vi "LIA Debugging Slow Host.vi"() -> ()   [LabVIEW 2017]
uses:
  Program Files (x86)/National Instruments/LabVIEW 2017/examples/Lock-In Amplifier/lib/host/Public/pll settings.ctl
  Program Files (x86)/National Instruments/LabVIEW 2017/examples/Lock-In Amplifier/lib/host/Public/lock-in settings.ctl
  Slow Class/LIA Debugging Slow.lvclass
  C:/Repositories/Lock-In-Amplifier/Debugging/Class/LIA Debugging.lvclass
  C:/Program Files (x86)/National Instruments/LabVIEW 2017/examples/Lock-In Amplifier/lib/interface/Interface/LIA Host Interface.lvclass
  <vilib>/measure/maspectr.llb/Power Spectrum and PSD Export Mode.ctl
  <vilib>/addons/Digital Filter Design/Analysis.llb/DFD Plot Freq Response (Linear-Spaced).vi
  <vilib>/measure/maspectr.llb/FFT Power Spectrum and PSD for N Chan.vi
  <vilib>/Utility/error.llb/Error Cluster From Error Code.vi
  <vilib>/rvi/errors/niLvFpgaAdjustHostInterfaceError.vi
  <vilib>/rvi/interface/nirviReadWriteControl/nirviReadWriteControl.xnode
  Program Files (x86)/National Instruments/LabVIEW 2017/examples/Lock-In Amplifier/lib/host/Lock-In Amplifier Example Host.lvlib
  Class/LIA Debugging.lvclass
  <vilib>/measure/NI_MAPro.lvlib
  <vilib>/addons/Digital Filter Design/NI_DigFilterLicensed.lvlib
  NiFpgaLv.dll
  <vilib>/rvi/interface/Simulation/niFpgaSimulationCallBeginRW.vi
  <vilib>/Analysis/4window.llb/windowTd.ctl
  <vilib>/Analysis/NI_AALPro.lvlib
  <vilib>/Analysis/NI_AALBase.lvlib
  <vilib>/measure/maspectr.llb/FFT Power Spectrum and PSD for 1 Chan (CDB).vi
panel:
  in  "Tab Control 2":enum32{"Page 1", "Page 2"}(tab)
  in  "restart averaging (F)":bool
  in  "dpll.m 0":i8=-20
  in  "lock-in.decimator0 0":enum16{"None", "CIC", "FIR", "2x4HB", "2x4SOS"}(ring)=enum."FIR"
  in  "averaging parameters":T1={"averaging mode"=enum."RMS averaging", "weighting mode"=enum."Exponential", "number of averages"=10} {"number of averages" min=1}
  in  "Host decimation?":bool
  in  "lock-in.iir config 0":T2={"b0"=0.001556396484375, "b1"=-0.000762939453125, "-a1"=1.9305267333984375, "-a2"=-0.9328765869140625} {"b0" format="%.17g"; "b1" format="%.17g"; "-a1" format="%.17g"; "-a2" format="%.17g"}
  out "lock-in.max-min":dbl=1.9775797561733533e-07 caption="Deviation" format="%#_6p"
  out "lock-in.min":dbl=1.9775797561733533e-07 caption="Deviation" format="%#_6p"
  out "lock-in.max":dbl=1.9775797561733533e-07 caption="Deviation" format="%#_6p"
  in  "Tab Control 1":T3(tab)
  out "pll.vco output 0":fxp<+/-,48,0> format="%#.18g"
  out "lock-in.cic config 0":cluster{"factor":fxp<+,16,16>, "shift":i16}
  out "dpll.vco output 0":fxp<+/-,48,0> format="%#.18g"
  out "dpll.config 0":T4
  out "nco.frequency 0":fxp<+/-,48,0>=0.0010000000000012221 format="%#_19g"
  out "stream.state 0":T5(ring)
  out "size(s) 1":i32
  out "lock-in.carrier 0 read":fxp<+/-,48,0> format="%_19g"
  out "stream.overflow? 0":bool
  out "size(s) 2":i32
  out "lock-in.decimator0 0 read":enum16{"None", "CIC", "FIR", "2x4HB", "2x4SOS"}(ring)
  out "size(s) 3":i32
  out "# elements in queue":i32
  out "Power Spectrum (dBm)":cluster{"f0":dbl, "df":dbl, "magnitude":dbl[]}[](graph)
  out "Waveform Graph 3":dbl[][](graph)
  out "Waveform Graph 4":dbl[][](graph)
  out "Waveform Graph 6":waveform(dbl)[](graph)
  out "Waveform Graph 2":cluster{"f0":dbl, "df":dbl, "values":dbl[]}[](graph)
  out "Waveform Graph":cluster{"f0":dbl, "df":dbl, "magnitude":dbl[]}[](graph)
  in  "app.quit":bool
  in  "lock-in.record length 0":u32=2048 caption="Record Length"
  in  "app.tab 0":enum32{"Lock-In", "PLL", "Output"}(tab)
  in  "lock-in.sampling rate":dbl=100000000.0 caption="Sampling Rate" format="%_10p"
  in  "lock-in.decimation0 0":i32=256 caption="Decimation 0"
  in  "lock-in.source 0":enum16{"AI 0", "AI 1", "AI 2", "AI 3", "NCO 0"}(ring)=enum."AI 1" caption="Channel"
  in  "lock-in.carrier 0":T6(ring)=enum."DPLL 0" caption="Carrier Source"
  in  "lock-in.manual carrier 0":dbl=100000.0 caption="Carrier Frequency" format="%_10p"
  in  "pll.source 0":enum16{"AI 0", "AI 1", "AI 2", "AI 3"}(ring) caption="Source"
  in  "pll.q frequency 0":dbl=100000.0 caption="Q Frequency" format="%#_6p"
  in  "pll.reset 0":bool caption="PLL Reset"
  in  "ao.level 0":dbl=0.5 caption="AO 0 Level" format="%#_6pV"
  in  "ao.frequency 0":dbl=10000000.0 caption="AO 0 Frequency" format="%#.9p"
  in  "rio device":tag="PXI2Slot2" caption="Resource"
  out "lock-in.deviation":dbl=1.9775797561733533e-07 caption="Deviation" format="%#_6p"
  out "lock-in.mean":dbl=8.221341747482856e-05 format="%#_12p"
  out "Result":cluster{dbl, "standard deviation":dbl}(graph)
  # "NI Lock-In Amplifier Reference Example"
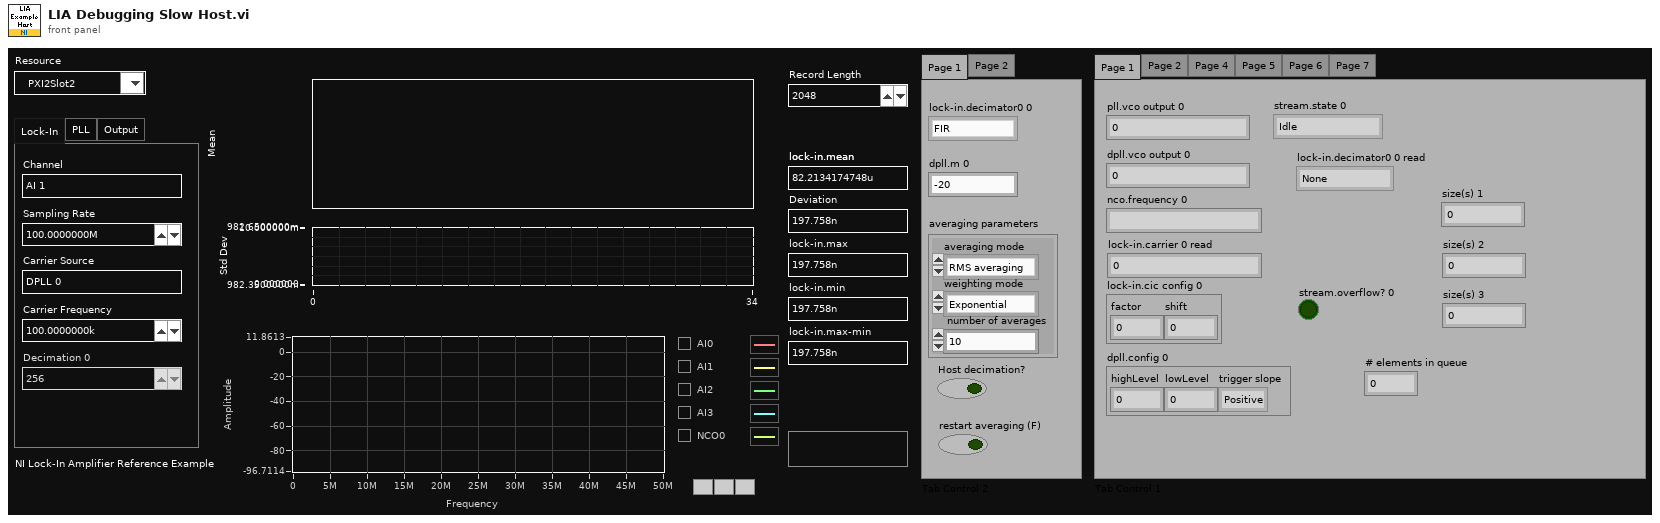
[diagram p1: front panel]
types:
  T1 = cluster{"averaging mode":enum16{"No averaging", "Vector averaging", "RMS averaging", "Peak hold"}, "weighting mode":enum16{"Linear", "Exponential"}, "number of averages":u32}
  T2 = cluster{"b0":fxp<+/-,18,2>, "b1":fxp<+/-,18,2>, "-a1":fxp<+/-,18,2>, "-a2":fxp<+/-,18,2>}
  T3 = enum32{"Page 1", "Page 2", "Page 4", "Page 5", "Page 6", "Page 7"}
  T4 = cluster{"highLevel":fxp<+/-,18,1>, "lowLevel":fxp<+/-,18,1>, "trigger slope":enum8{"Positive", "Negative"}}
  T5 = enum8{"Idle", "Finite Transfer", "Continuous", "Done", "Error", "Not Ready", "Cancel"}
  T6 = enum16{"Manual 0", "Manual 1", "Manual 2", "Manual 3", "PLL 0", "PLL 1", "DPLL 0", "DPLL 1"}
  T7 = typedef "Lock-In Amplifier Example Host.lvlib/lock-in settings.ctl" = cluster{"decimation":i32, "source":i32, "carrier source":i32, "carrier":dbl}
  T8 = typedef "Lock-In Amplifier Example Host.lvlib/pll settings.ctl" = cluster{"source":i32, "q frequency":dbl}
  T9 = typedef "NI_DigFilterLicensed.lvlib/DFD Filter Obj.ctl" = cluster{"mSRate_Fs":dbl, "mSRate_Version":string, "mSRate_Comments":string, "mSRate_OrgCoef":T10, "mSRate_CurCoef":T10, "mSRate_Quantized?":bool, "mSRate_QCoef":T10, "mSRate_QSettings":T12[], "mSRate_Order":i32, "mSRate_Scaling":cluster{"mSRate_ScaleByPowerOf2?":bool, "mSRate_ScaleType":T14}}
  T10 = typedef "NI_DigFilterLicensed.lvlib/DFD Filter Coef.ctl" = cluster{"type":T11, "gain":dbl, "coef a (k)":dbl[], "coef b (v)":dbl[]}
  T11 = typedef "NI_DigFilterLicensed.lvlib/DFD Filter Structure Type Selector.ctl" = enum16{"Undefined", "FIR Direct Form", "FIR Direct Form Transposed", "FIR Symmetric", "FIR Antisymmetric", "IIR Direct Form I", "IIR Direct Form I Transposed", "IIR Direct Form II", "IIR Direct Form II Transposed", "IIR Cascaded Second Order Sections Form I", "IIR Cascaded Second Order Sections Form I Transposed", "IIR Cascaded Second Order Sections Form II", "IIR Cascaded Second Order Sections Form II Transposed", "Lattice Allpass (basic sections)", "Lattice Allpass (one multiplier sections)", "Lattice Allpass (normalized sections)", "Lattice AR (basic sections)", "Lattice AR (one multiplier sections)", "Lattice AR (normalized sections)", "Lattice MA (minimum phase)", "Lattice MA (maximum phase)", "Lattice ARMA (basic sections)", "Lattice ARMA (one multiplier sections)", "Lattice ARMA (normalized sections)"}
  T12 = typedef "NI_DigFilterLicensed.lvlib/dfd_Internal Quantization Settings.ctl" = cluster{"source":T13, "wl":i16, "iwl":i16, "overflow mode":enum16{"Saturation", "Wrap"}, "rounding mode":enum16{"Nearest", "Truncation"}, "signed?":bool}
  T13 = typedef "NI_DigFilterLicensed.lvlib/dfd_Internal Quantization Srcs.ctl" = u16
  T14 = typedef "NI_DigFilterLicensed.lvlib/DFD Coef Norm Type.ctl" = enum16{"No Norm", "Time Domain 1-Norm", "Time Domain 2-Norm", "Time Domain Inf-Norm"}
  T15 = cluster{"t0":dbl, "dt":dbl, "amplitudes":dbl[]}[]
  T16 = typedef "NI_MAPro.lvlib/Power Spectrum and PSD Export Mode.ctl" = u16
  T17 = typedef "NI_AALPro.lvlib/windowTd.ctl" = u32
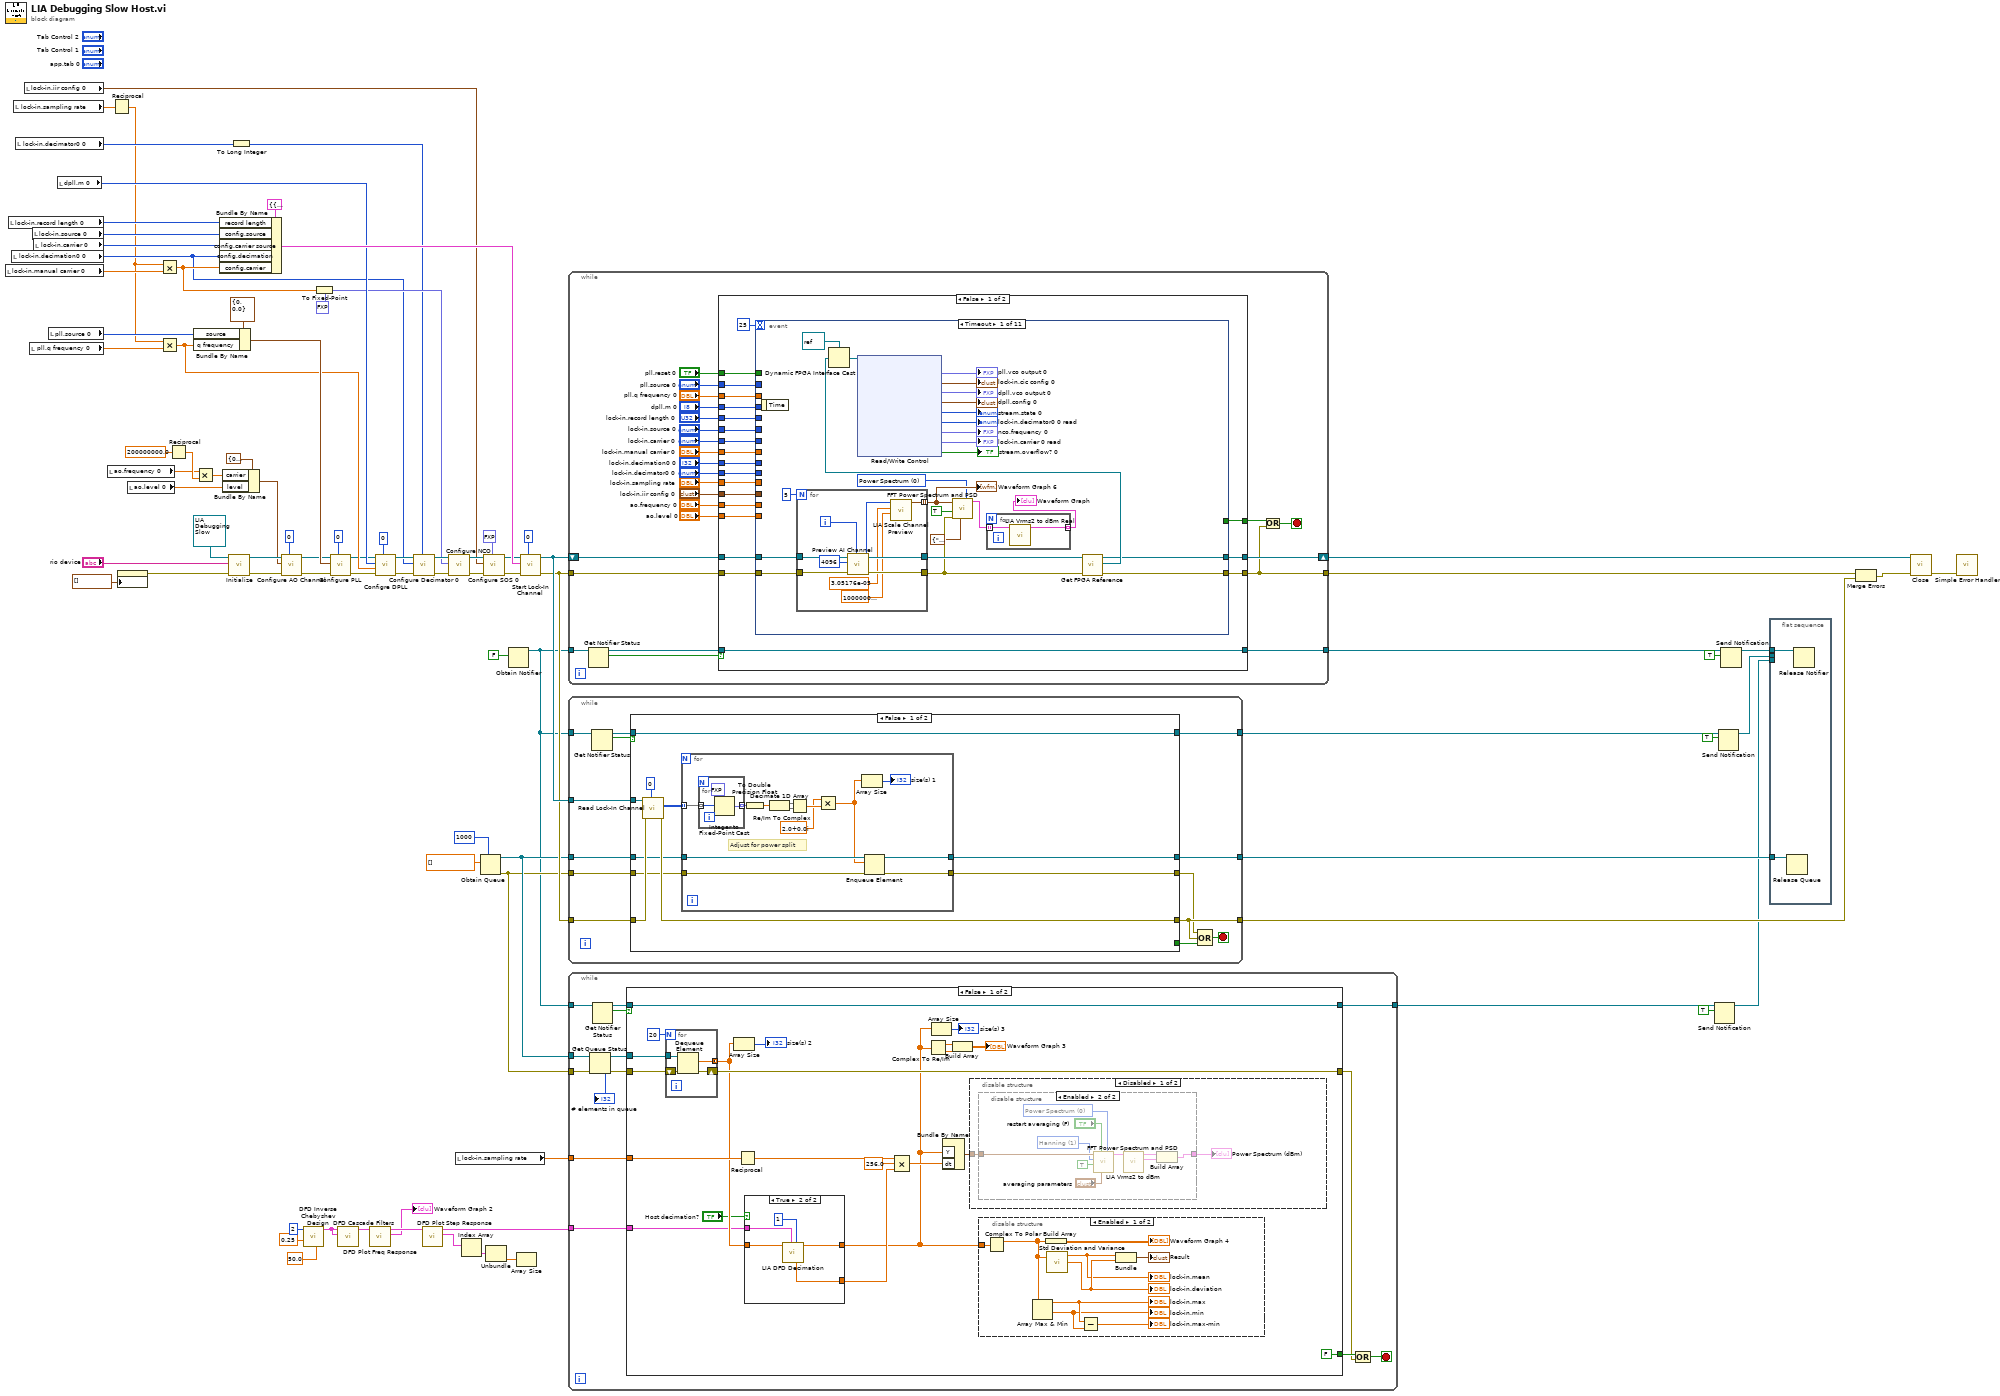
[diagram p0: block diagram]
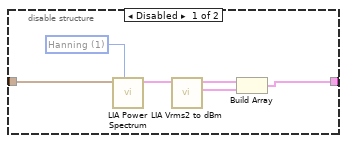
[diagram p2: hidden frame]
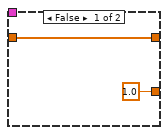
[diagram p4: hidden frame]
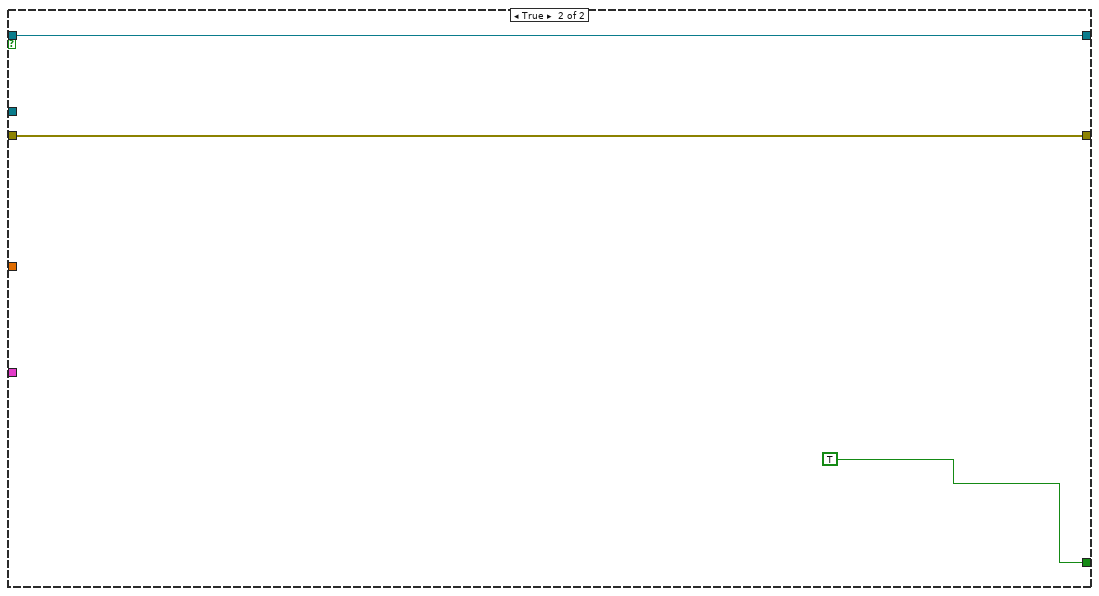
[diagram p6: hidden frame]
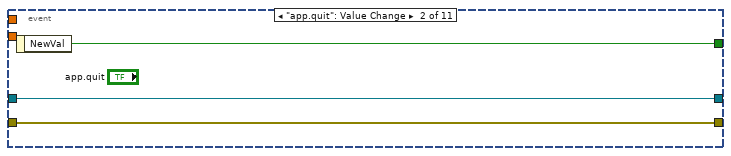
[diagram p7: hidden frame]
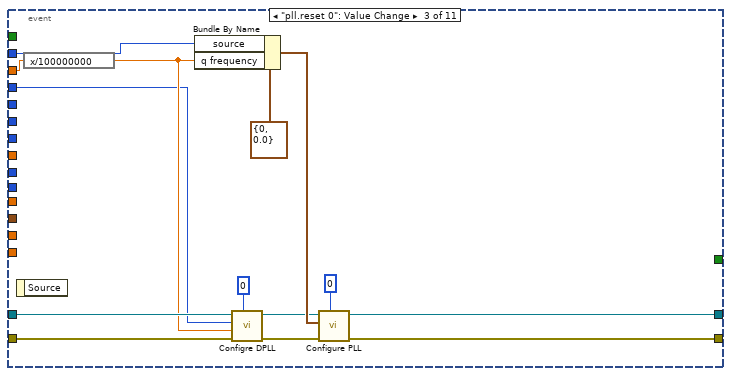
[diagram p8: hidden frame]
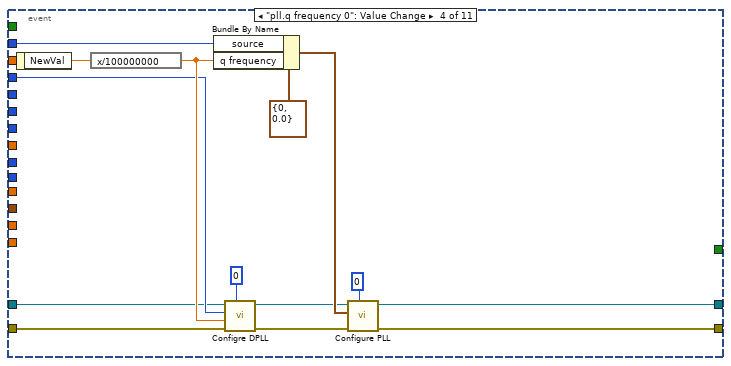
[diagram p9: hidden frame]
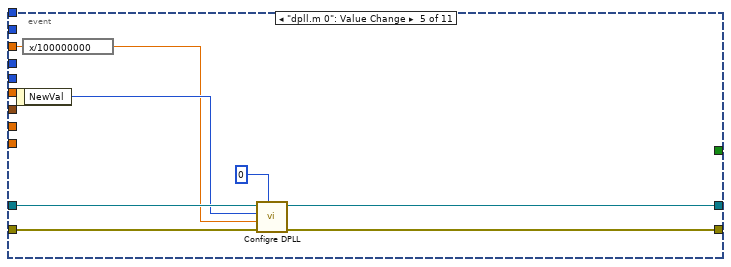
[diagram p10: hidden frame]
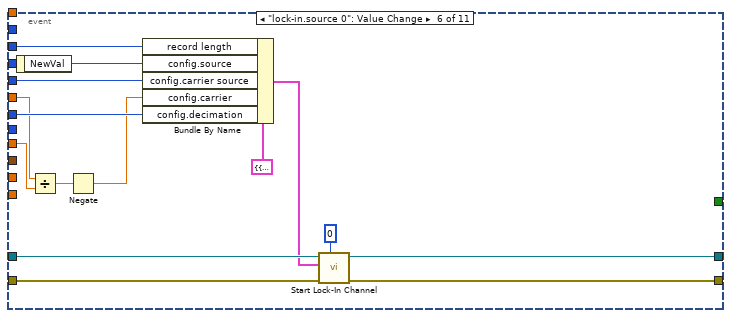
[diagram p11: hidden frame]
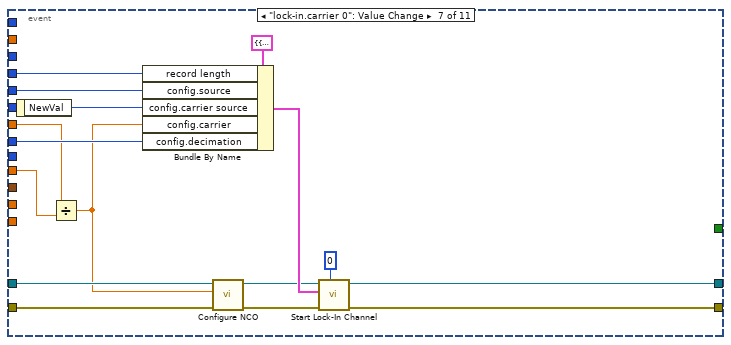
[diagram p12: hidden frame]
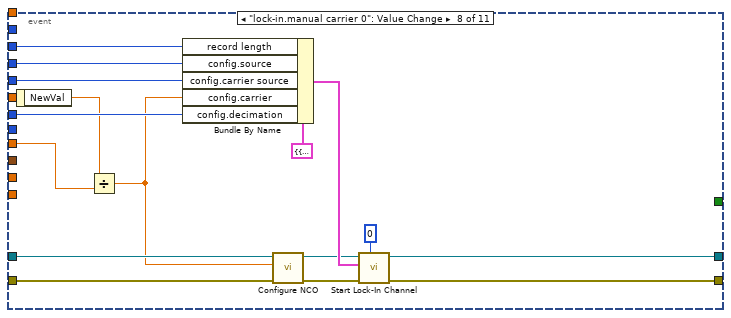
[diagram p13: hidden frame]
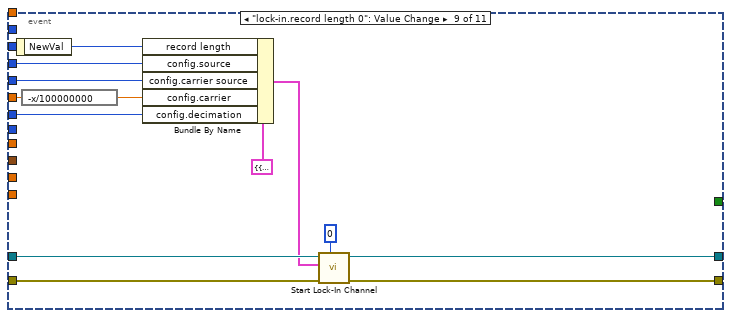
[diagram p14: hidden frame]
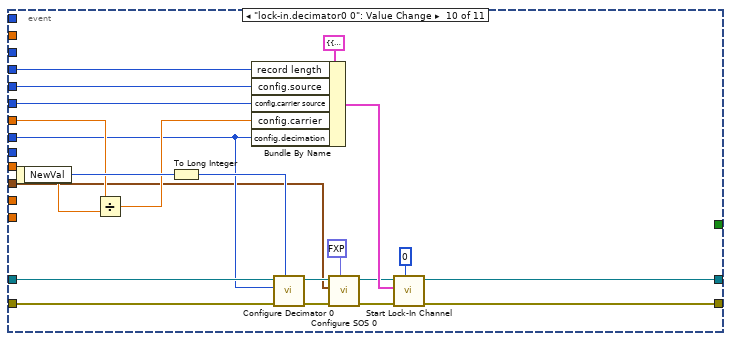
[diagram p15: hidden frame]
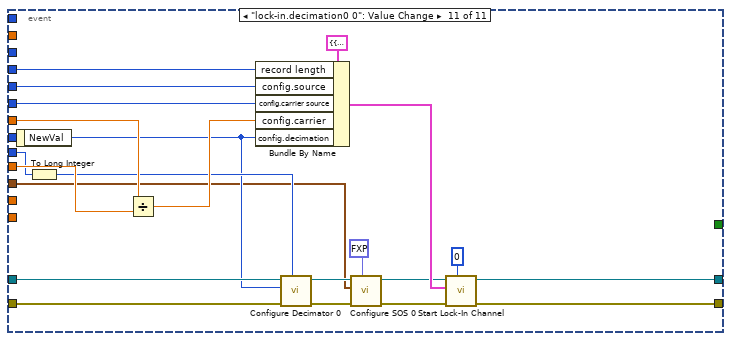
[diagram p16: hidden frame]
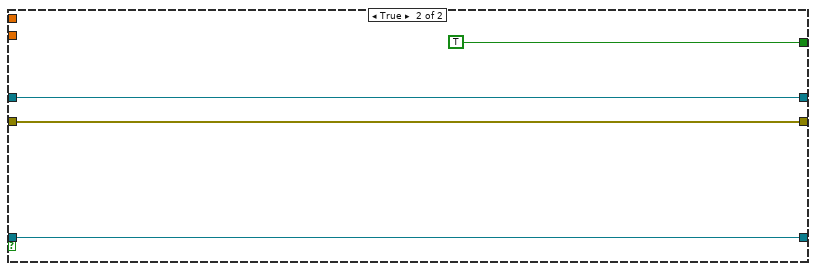
[diagram p17: hidden frame]
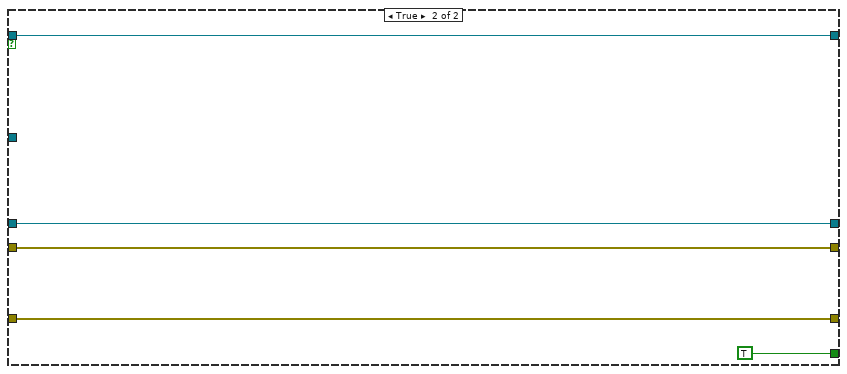
[diagram p18: hidden frame]
diagram:
  n1 = local read "lock-in.manual carrier 0"() -> (w81:dbl)
  n2 = local read "lock-in.record length 0"() -> (w65:u32)
  n3 = local read "lock-in.decimation0 0"() -> (w37:i32)
  n4 = local read "lock-in.sampling rate"() -> (w53:dbl)
  n5 = local read "lock-in.decimator0 0"() -> (w49:enum16{"None", "CIC", "FIR", "2x4HB", "2x4SOS"})
  n6 = local read "lock-in.iir config 0"() -> (w35:T2)
  n7 = local read "pll.q frequency 0"() -> (w82:dbl)
  n8 = local read "lock-in.source 0"() -> (w86:enum16{"AI 0", "AI 1", "AI 2", "AI 3", "NCO 0"})
  n9 = local read "lock-in.carrier 0"() -> (w85:T6)
  n10 = local read "pll.source 0"() -> (w83:enum16{"AI 0", "AI 1", "AI 2", "AI 3"})
  n11 = local read "dpll.m 0"() -> (w60:i8)
  n12 = local read "ao.frequency 0"() -> (w9:dbl)
  n13 = Reciprocal(x=w53) -> (1/x=w33:dbl)
  n14 = property on="Result" class="WFChart (strict)"("History Data"=cluster{dbl, "standard deviation":dbl}[] []) -> (error out=w40:errorcluster)  [unwired: 2 in, 1 out]
  n15 = local read "ao.level 0"() -> (w8:dbl)
  n16 = Multiply(x=w33, y=w81) -> (x*y=w42:dbl)
  n17 = Multiply(x=w33, y=w82) -> (x*y=w56:dbl)
  n18 = Reciprocal(x=200000000.0) -> (1/x=w17:dbl)
  n19 = Bundle By Name(cluster=T8 {"source"=0, "q frequency"=0.0} ("config"), "source"=w83, "q frequency"=w56) -> (w57:T8)
  n20 = Multiply(x=w9, y=w17) -> (x*y=w18:dbl)
  n21 = Bundle By Name(cluster=cluster{"config":T7, "record length":u32} {"config"={"decimation"=0, "source"=0, "carrier source"=0, "carrier"=0.0}, "record length"=0} ("config"), "record length"=w65, "config.source"=w86, "config.carrier source"=w85, "config.decimation"=w37, "config.carrier"=w42) -> (w66:cluster{"config":T7, "record length":u32})
  n22 = Bundle By Name(cluster=cluster{"carrier":dbl, "level":dbl} {"carrier"=0.0, "level"=0.0} ("config"), "carrier"=w18, "level"=w8) -> (w7:cluster{"carrier":dbl, "level":dbl})
  n23 = call-dynamic "Initialize.vi"("error in"=w40, "resource"="rio device", "host in"=refnum<class "LIA Debugging Slow.lvclass"> refnum ("LIA Debugging Slow.lvclass")) -> ("error out"=w13:errorcluster, "host out"=w15:refnum<class "LIA Debugging Slow.lvclass">)  [unwired: 7 in]
  n24 = To Long Integer(number=w49) -> (32bit integer=w38:i32)
  n25 = call-dynamic "Configure AO Channel.vi"("index"=0, "error in"=w13, "config"=w7, "host in"=w15) -> ("error out"=w12:errorcluster, "host out"=w14:refnum<class "LIA Debugging Slow.lvclass">)  [unwired: 6 in]
  n26 = call <vilib>:"DFD Inverse Chebyshev Design.vi"("stopband atten [dB]"=50.0, "low cutoff freq [Hz]"=0.25, "order"=2) -> ("filter out"=w30:T9)  [unwired: 7 in, 1 out]
  n27 = To Fixed-Point(fixed-point type=fxp<+/-,48,0> 0.0 ("nco.frequency 0"), number=w42) -> (fixed-point=w55:fxp<+/-,48,0>)
  n28 = call-dynamic "Configure PLL.vi"("index"=0, "error in"=w12, "config"=w57, "host in"=w14) -> ("error out"=w47:errorcluster, "host out"=w48:refnum<class "LIA Debugging Slow.lvclass">)  [unwired: 6 in]
  n29 = call <vilib>:"DFD Cascade Filters.vi"("filter in 2"=w30, "filter in 1"=w30) -> ("filter out"=w5:T9)  [unwired: 8 in, 1 out]
  n30 = call-poly <vilib>:"DFD Plot Freq Response.vi"("filter in"=w5) -> ("magnitude response"=→"Waveform Graph 2":cluster{"f0":dbl, "df":dbl, "values":dbl[]}[], "filter out"=w21:T9)  [unwired: 7 in, 2 out]
  n31 = call "Configre DPLL.vi"("dpll.channel 0"=0, "error in (no error)"=w47, "dpll.q 0"=w56, "dpll.m 0"=w60, "LIA Host Interface in"=w48) -> ("error out"=w61:errorcluster, "LIA Host Interface Out"=w62:refnum<class "LIA Debugging Slow.lvclass">)  [unwired: 5 in]
  n32 = call-dynamic "Configure Decimator 0.vi"("lock-in.decimator0 0"=w38, "error in (no error)"=w61, "lock-in.decimation0 0"=w37, "LIA Host Interface in"=w62) -> ("error out"=w58:errorcluster, "LIA Host Interface out"=w59:refnum<class "LIA Debugging Slow.lvclass">)  [unwired: 6 in]
  n33 = call <vilib>:"DFD Plot Step Response.vi"("filter in"=w21) -> ("step response"=w29:T15, "filter out"=w20:T9)  [unwired: 8 in, 1 out]
  n34 = call "Configure NCO.vi"("error in (no error)"=w58, "nco.frequency 0"=w55, "LIA Host Interface in"=w59) -> ("error out"=w50:errorcluster, "LIA Host Interface out"=w51:refnum<class "LIA Debugging Slow.lvclass">)  [unwired: 7 in]
  n35 = local read "lock-in.sampling rate"() -> (w22:dbl)
  n36 = Index Array(array=w29) -> (element=w28:cluster{"t0":dbl, "dt":dbl, "amplitudes":dbl[]})  [unwired: 1 in]
  n37 = Obtain Queue(max queue size (-1, unlimited)=1000, element data type=cdb[] [] ("x + iy")) -> (queue out=w25:refnum<queue>, error out=w24:errorcluster)  [unwired: 3 in, 1 out]
  n38 = call "Configure SOS 0.vi"("lock-in.iir decimation0 0"=fxp<+,4,4> 1.0, "error in (no error)"=w50, "lock-in.iir config 0 0"=w35, "LIA Host Interface in"=w51) -> ("error out"=w44:errorcluster, "LIA Host Interface out"=w46:refnum<class "LIA Debugging Slow.lvclass">)  [unwired: 6 in]
  n39 = Unbundle(w28) -> ("amplitudes"=w19:dbl[])  [unwired: 2 out]
  n40 = Obtain Notifier(notification data type=FALSE) -> (notifier out=w23:refnum<notifier>)  [unwired: 3 in, 2 out]
  n41 = Array Size(array=w19) -> ()  [unwired: 1 out]
  n42 = call-dynamic "Start Lock-In Channel.vi"("index"=0, "error in"=w44, "config"=w66, "host in"=w46) -> ("error out"=w43:errorcluster, "host out"=w45:refnum<class "LIA Debugging Slow.lvclass">)  [unwired: 6 in]
  n43 = while {
    tunnel: w43 -> [w110]
    shift-right: [w102] -> w80
    shift-left: w45 -> [w109]
    tunnel: [w98] -> w71
    tunnel: w23 -> [w101]
    tunnel: [w96] -> w78
    stop <- w108 stop-if-true
    n44 = Get Notifier Status(notifier=w101) -> (notifier out=w100:refnum<notifier>, current notification=w99:bool)  [unwired: 1 in, 3 out]
    n45 = case shown="False" w99 {
      tunnel: w110 -> [w131 w314]
      tunnel: w109 -> [w130 w315]
      tunnel: [w129 w314] -> w98
      tunnel: "lock-in.manual carrier 0" -> [w127 _]
      tunnel: "lock-in.decimation0 0" -> [w126 _]
      tunnel: "lock-in.source 0" -> [w125 _]
      tunnel: "lock-in.carrier 0" -> [w124 _]
      tunnel: "pll.source 0" -> [w123 _]
      tunnel: "pll.q frequency 0" -> [w122 _]
      tunnel: [w121 w315] -> w102
      tunnel: w100 -> [w119 w312]
      tunnel: [w120 TRUE] -> w97
      tunnel: [w119 w312] -> w96
      tunnel: "lock-in.record length 0" -> [w118 _]
      tunnel: "dpll.m 0" -> [w117 _]
      tunnel: "lock-in.decimator0 0" -> [w116 _]
      tunnel: "lock-in.sampling rate" -> [w115 _]
      tunnel: "pll.reset 0" -> [w114 _]
      tunnel: "lock-in.iir config 0" -> [w113 _]
      tunnel: "ao.frequency 0" -> [w112 _]
      tunnel: "ao.level 0" -> [w111 _]
      frame False {
        n46 = event shown="[0] Timeout" {
          selector: _ -> [_ _ _ _ _ _ _ _ _ _ _]
          dyn-events: _ -> [_ _ _ _ _ _ _ _ _ _ _]
          timeout: 25 -> [_ _ _ _ _ _ _ _ _ _ _]
          tunnel: w131 -> [w155 w170 w175 w186 w202 w220 w228 w241 w263 w281 w303]
          tunnel: w130 -> [w156 w171 w177 w187 w207 w218 w230 w243 w261 w282 w304]
          tunnel: [w152 w170 w185 w195 w200 w219 w237 w252 w262 w280 w302] -> w129
          tunnel: w125 -> [_ _ _ _ _ _ w231 w246 w255 w286 w308]
          tunnel: w124 -> [_ _ _ _ _ w222 _ w254 w266 w289 w311]
          tunnel: w127 -> [_ _ _ _ w204 w210 w225 _ w265 w277 w300]
          tunnel: w126 -> [_ _ _ _ _ w221 w238 w253 w264 w274 _]
          tunnel: w123 -> [_ _ w182 w198 _ _ _ _ _ _ _]
          tunnel: w122 -> [_ _ w179 _ _ _ _ _ _ _ _]
          tunnel: [w140 w171 w180 w196 w201 w217 w223 w251 w260 w288 w310] -> w121
          tunnel: [_ w169 _ _ _ _ _ _ _ _ _] -> w120
          tunnel: w118 -> [_ _ _ _ _ w214 w234 w248 _ w284 w306]
          tunnel: w117 -> [_ _ w172 w190 _ _ _ _ _ _ _]
          tunnel: w116 -> [_ _ _ _ _ _ _ _ _ _ w299]
          tunnel: w115 -> [_ _ _ _ _ w209 w226 w244 _ w278 w301]
          tunnel: w114 -> [_ _ _ _ _ _ _ _ _ _ _]
          tunnel: w113 -> [_ _ _ _ _ _ _ _ _ w268 w292]
          tunnel: w112 -> [_ _ _ _ _ _ _ _ _ _ _]
          tunnel: w111 -> [_ _ _ _ _ _ _ _ _ _ _]
          event Timeout {
            w135 = T16 0 items=["Power Spectrum", "Power Spectral Density"] ("export mode")
            n47 = event-data() -> ()  [unwired: 1 in, 1 out]
            n48 = for {
              N: 5 -> [_]
              tunnel: w156 -> [w168]
              tunnel: [w166] -> w153
              tunnel: w155 -> [w167]
              tunnel: [w164] -> w144
              tunnel: [w162] -> w142 mode=indexing
              i -> [w159]
              n49 = call-dynamic "Preview AI Channel.vi"("index"=w159, "error in"=w167, "samples"=u32 4096, "host in"=w168) -> ("error out"=w164:errorcluster, "samples out"=w163:i16[], "host out"=w166:refnum<class "LIA Debugging Slow.lvclass">)  [unwired: 5 in]
              n50 = call "LIA Scale Channel Preview.vi"("sample rate"=100000000.0, "scaling factor"=3.05176e-05, "ai data"=w163) -> ("Waveform"=w162:waveform(dbl))  [unwired: 8 in]
            }
            "Waveform Graph 6" <- w142
            n51 = call-poly <vilib>:"FFT Power Spectrum and PSD.vi"("export mode"=w135, "averaging parameters"=T1 {"averaging mode"=enum."RMS averaging", "weighting mode"=enum."Exponential", "number of averages"=10}, "error in (no error)"=w144, "dB On (F)"=TRUE, "time signals"=w142) -> ("Power Spectrum / PSD"=w134:cluster{"f0":dbl, "df":dbl, "magnitude":dbl[]}[])  [unwired: 3 in, 3 out]
            n52 = for {
              tunnel: w134 -> [w158] mode=indexing
              tunnel: [w157] -> w133 mode=indexing
              n53 = call "LIA Vrms2 to dBm Real.vi"("Power Spectrum / PSD"=w158) -> ("Power Spectrum / PSD (dBm)"=w157:cluster{"f0":dbl, "df":dbl, "magnitude":dbl[]})  [unwired: 9 in, 1 out]
            }
            "Waveform Graph" <- w133
            n54 = call "Get FPGA Reference.vi"("error in (no error)"=w144, "LIA Host Interface in"=w153) -> ("error out"=w152:errorcluster, "Properties:FPGA Session"=w151:refnum<k20>, "LIA Host Interface out"=w140:refnum<class "LIA Debugging Slow.lvclass">)  [unwired: 7 in]
            n55 = Dynamic FPGA Interface Cast(Session In=refnum<k20> refnum ("fpga type"), Type=w151) -> (Session Out=w149:refnum<k20>)
            n56 = xnode "Read/Write Control"("FPGA VI Reference In"=w149) -> ("pll.vco output 0"=→"pll.vco output 0":fxp<+/-,48,0>, "lock-in.cic config 0"=→"lock-in.cic config 0":cluster{"factor":fxp<+,16,16>, "shift":i16}, "dpll.vco output 0"=→"dpll.vco output 0":fxp<+/-,48,0>, "dpll.config 0"=→"dpll.config 0":T4, "stream.state 0"=→"stream.state 0":T5, "lock-in.decimator0 0"=→"lock-in.decimator0 0 read":enum16{"None", "CIC", "FIR", "2x4HB", "2x4SOS"}, "nco.frequency 0"=→"nco.frequency 0":fxp<+/-,48,0>, "lock-in.carrier 0"=→"lock-in.carrier 0 read":fxp<+/-,48,0>, "stream.overflow? 0"=→"stream.overflow? 0":bool)  [unwired: 1 in, 2 out]
          }
          event "app.quit": Value Change {
            n57 = event-data() -> ("NewVal"=w169:bool)  [unwired: 1 in]
          }
          event "pll.reset 0": Value Change {
            n58 = event-data() -> ()  [unwired: 1 in, 1 out]
            n59 = expression code="x/100000000"(w179) -> (w173:dbl)
            n60 = Bundle By Name(cluster=T8 {"source"=0, "q frequency"=0.0} ("config"), "source"=w182, "q frequency"=w173) -> (w181:T8)
            n61 = call "Configre DPLL.vi"("dpll.channel 0"=0, "error in (no error)"=w175, "dpll.q 0"=w173, "dpll.m 0"=w172, "LIA Host Interface in"=w177) -> ("error out"=w174:errorcluster, "LIA Host Interface Out"=w176:refnum<class "LIA Debugging Slow.lvclass">)  [unwired: 5 in]
            n62 = call-dynamic "Configure PLL.vi"("index"=0, "error in"=w174, "config"=w181, "host in"=w176) -> ("error out"=w185:errorcluster, "host out"=w180:refnum<class "LIA Debugging Slow.lvclass">)  [unwired: 6 in]
          }
          event "pll.q frequency 0": Value Change {
            n63 = event-data() -> ("NewVal"=w197:dbl)  [unwired: 1 in]
            n64 = expression code="x/100000000"(w197) -> (w191:dbl)
            n65 = Bundle By Name(cluster=T8 {"source"=0, "q frequency"=0.0} ("config"), "source"=w198, "q frequency"=w191) -> (w194:T8)
            n66 = call "Configre DPLL.vi"("dpll.channel 0"=0, "error in (no error)"=w186, "dpll.q 0"=w191, "dpll.m 0"=w190, "LIA Host Interface in"=w187) -> ("error out"=w188:errorcluster, "LIA Host Interface Out"=w189:refnum<class "LIA Debugging Slow.lvclass">)  [unwired: 5 in]
            n67 = call-dynamic "Configure PLL.vi"("index"=0 ("instance"), "error in"=w188, "config"=w194, "host in"=w189) -> ("error out"=w195:errorcluster, "host out"=w196:refnum<class "LIA Debugging Slow.lvclass">)  [unwired: 6 in]
          }
          event "dpll.m 0": Value Change {
            n68 = event-data() -> ("NewVal"=w205:i8)  [unwired: 1 in]
            n69 = expression code="x/100000000"(w204) -> (w203:dbl)
            n70 = call "Configre DPLL.vi"("dpll.channel 0"=0, "error in (no error)"=w202, "dpll.q 0"=w203, "dpll.m 0"=w205, "LIA Host Interface in"=w207) -> ("error out"=w200:errorcluster, "LIA Host Interface Out"=w201:refnum<class "LIA Debugging Slow.lvclass">)  [unwired: 5 in]
          }
          event "lock-in.source 0": Value Change {
            n71 = event-data() -> ("NewVal"=w212:enum16{"AI 0", "AI 1", "AI 2", "AI 3", "NCO 0"})  [unwired: 1 in]
            n72 = Divide(x=w210, y=w209) -> (x/y=w211:dbl)
            n73 = Negate(x=w211) -> (-x=w208:dbl)
            n74 = Bundle By Name(cluster=cluster{"config":T7, "record length":u32} {"config"={"decimation"=0, "source"=0, "carrier source"=0, "carrier"=0.0}, "record length"=0} ("config"), "record length"=w214, "config.source"=w212, "config.carrier source"=w222, "config.carrier"=w208, "config.decimation"=w221) -> (w213:cluster{"config":T7, "record length":u32})
            n75 = call-dynamic "Start Lock-In Channel.vi"("index"=0, "error in"=w220, "config"=w213, "host in"=w218) -> ("error out"=w219:errorcluster, "host out"=w217:refnum<class "LIA Debugging Slow.lvclass">)  [unwired: 6 in]
          }
          event "lock-in.carrier 0": Value Change {
            n76 = event-data() -> ("NewVal"=w232:T6)  [unwired: 1 in]
            n77 = Divide(x=w225, y=w226) -> (x/y=w224:dbl)
            n78 = Bundle By Name(cluster=cluster{"config":T7, "record length":u32} {"config"={"decimation"=0, "source"=0, "carrier source"=0, "carrier"=0.0}, "record length"=0} ("config"), "record length"=w234, "config.source"=w231, "config.carrier source"=w232, "config.carrier"=w224, "config.decimation"=w238) -> (w233:cluster{"config":T7, "record length":u32})
            n79 = call "Configure NCO.vi"("error in (no error)"=w228, "nco.frequency 0"=w224, "LIA Host Interface in"=w230) -> ("error out"=w227:errorcluster, "LIA Host Interface out"=w229:refnum<class "LIA Debugging Slow.lvclass">)  [unwired: 7 in]
            n80 = call-dynamic "Start Lock-In Channel.vi"("index"=0, "error in"=w227, "config"=w233, "host in"=w229) -> ("error out"=w237:errorcluster, "host out"=w223:refnum<class "LIA Debugging Slow.lvclass">)  [unwired: 6 in]
          }
          event "lock-in.manual carrier 0": Value Change {
            n81 = event-data() -> ("NewVal"=w245:dbl)  [unwired: 1 in]
            n82 = Divide(x=w245, y=w244) -> (x/y=w239:dbl)
            n83 = Bundle By Name(cluster=cluster{"config":T7, "record length":u32} {"config"={"decimation"=0, "source"=0, "carrier source"=0, "carrier"=0.0}, "record length"=0} ("config"), "record length"=w248, "config.source"=w246, "config.carrier source"=w254, "config.carrier"=w239, "config.decimation"=w253) -> (w247:cluster{"config":T7, "record length":u32})
            n84 = call "Configure NCO.vi"("error in (no error)"=w241, "nco.frequency 0"=w239, "LIA Host Interface in"=w243) -> ("error out"=w240:errorcluster, "LIA Host Interface out"=w242:refnum<class "LIA Debugging Slow.lvclass">)  [unwired: 7 in]
            n85 = call-dynamic "Start Lock-In Channel.vi"("index"=0, "error in"=w240, "config"=w247, "host in"=w242) -> ("error out"=w252:errorcluster, "host out"=w251:refnum<class "LIA Debugging Slow.lvclass">)  [unwired: 6 in]
          }
          event "lock-in.record length 0": Value Change {
            n86 = event-data() -> ("NewVal"=w256:u32)  [unwired: 1 in]
            n87 = expression code="-x/100000000"(w265) -> (w267:dbl)
            n88 = Bundle By Name(cluster=cluster{"config":T7, "record length":u32} {"config"={"decimation"=0, "source"=0, "carrier source"=0, "carrier"=0.0}, "record length"=0} ("config"), "record length"=w256, "config.source"=w255, "config.carrier source"=w266, "config.carrier"=w267, "config.decimation"=w264) -> (w257:cluster{"config":T7, "record length":u32})
            n89 = call-dynamic "Start Lock-In Channel.vi"("index"=0, "error in"=w263, "config"=w257, "host in"=w261) -> ("error out"=w262:errorcluster, "host out"=w260:refnum<class "LIA Debugging Slow.lvclass">)  [unwired: 6 in]
          }
          event "lock-in.decimator0 0": Value Change {
            n90 = event-data() -> ("NewVal"=w279:enum16{"None", "CIC", "FIR", "2x4HB", "2x4SOS"})  [unwired: 1 in]
            n91 = Divide(x=w277, y=w278) -> (x/y=w276:dbl)
            n92 = To Long Integer(number=w279) -> (32bit integer=w275:i32)
            n93 = Bundle By Name(cluster=cluster{"config":T7, "record length":u32} {"config"={"decimation"=0, "source"=0, "carrier source"=0, "carrier"=0.0}, "record length"=0} ("config"), "record length"=w284, "config.source"=w286, "config.carrier source"=w289, "config.carrier"=w276, "config.decimation"=w274) -> (w283:cluster{"config":T7, "record length":u32})
            n94 = call-dynamic "Configure Decimator 0.vi"("lock-in.decimator0 0"=w275, "error in (no error)"=w281, "lock-in.decimation0 0"=w274, "LIA Host Interface in"=w282) -> ("error out"=w271:errorcluster, "LIA Host Interface out"=w272:refnum<class "LIA Debugging Slow.lvclass">)  [unwired: 6 in]
            n95 = call "Configure SOS 0.vi"("lock-in.iir decimation0 0"=fxp<+,4,4> 1.0, "error in (no error)"=w271, "lock-in.iir config 0 0"=w268, "LIA Host Interface in"=w272) -> ("error out"=w269:errorcluster, "LIA Host Interface out"=w270:refnum<class "LIA Debugging Slow.lvclass">)  [unwired: 6 in]
            n96 = call-dynamic "Start Lock-In Channel.vi"("index"=0, "error in"=w269, "config"=w283, "host in"=w270) -> ("error out"=w280:errorcluster, "host out"=w288:refnum<class "LIA Debugging Slow.lvclass">)  [unwired: 6 in]
          }
          event "lock-in.decimation0 0": Value Change {
            n97 = event-data() -> ("NewVal"=w296:i32)  [unwired: 1 in]
            n98 = To Long Integer(number=w299) -> (32bit integer=w297:i32)
            n99 = Divide(x=w300, y=w301) -> (x/y=w298:dbl)
            n100 = Bundle By Name(cluster=cluster{"config":T7, "record length":u32} {"config"={"decimation"=0, "source"=0, "carrier source"=0, "carrier"=0.0}, "record length"=0} ("config"), "record length"=w306, "config.source"=w308, "config.carrier source"=w311, "config.carrier"=w298, "config.decimation"=w296) -> (w305:cluster{"config":T7, "record length":u32})
            n101 = call-dynamic "Configure Decimator 0.vi"("lock-in.decimator0 0"=w297, "error in (no error)"=w303, "lock-in.decimation0 0"=w296, "LIA Host Interface in"=w304) -> ("error out"=w293:errorcluster, "LIA Host Interface out"=w294:refnum<class "LIA Debugging Slow.lvclass">)  [unwired: 6 in]
            n102 = call "Configure SOS 0.vi"("lock-in.iir decimation0 0"=fxp<+,4,4> 1.0, "error in (no error)"=w293, "lock-in.iir config 0 0"=w292, "LIA Host Interface in"=w294) -> ("error out"=w290:errorcluster, "LIA Host Interface out"=w291:refnum<class "LIA Debugging Slow.lvclass">)  [unwired: 6 in]
            n103 = call-dynamic "Start Lock-In Channel.vi"("index"=0, "error in"=w290, "config"=w305, "host in"=w291) -> ("error out"=w302:errorcluster, "host out"=w310:refnum<class "LIA Debugging Slow.lvclass">)  [unwired: 6 in]
          }
        }
      }
      frame True {
      }
    }
    n104 = Or(x=w97, y=w98) -> (x .or. y?=w108:bool)
  }
  n105 = while {
    tunnel: w23 -> [w328]
    tunnel: w45 -> [w325]
    tunnel: w43 -> [w324]
    tunnel: [w323] -> w72
    tunnel: [w320] -> w75
    tunnel: w25 -> [w319]
    tunnel: [w318] -> w26
    tunnel: w24 -> [w317]
    stop <- w322 stop-if-true
    n106 = Get Notifier Status(notifier=w328) -> (notifier out=w326:refnum<notifier>, current notification=w327:bool)  [unwired: 1 in, 3 out]
    n107 = case shown="False" w327 {
      tunnel: [w335 w359] -> w320
      tunnel: w326 -> [w335 w359]
      tunnel: w325 -> [w338 _]
      tunnel: w324 -> [w337 w358]
      tunnel: [w334 w358] -> w323
      tunnel: [_ TRUE] -> w321
      tunnel: w319 -> [w332 w356]
      tunnel: [w331 w356] -> w318
      tunnel: w317 -> [w330 w355]
      tunnel: [w329 w355] -> w316
      frame False {
        n108 = call-dynamic "Read Lock-In Channel.vi"("index"=0, "error in"=w337, "host in"=w338) -> ("error out"=w334:errorcluster, "unscaled data"=w333:i64[][])  [unwired: 6 in, 1 out]
        n109 = for {
          tunnel: w333 -> [w346] mode=indexing
          tunnel: w332 -> [w343]
          tunnel: [w342] -> w331
          tunnel: w330 -> [w345]
          tunnel: [w344] -> w329
          # "Adjust for power split"
          n110 = for {
            tunnel: w346 -> [w354] mode=indexing
            tunnel: [w352] -> w348 mode=indexing
            n111 = Integer to Fixed-Point Cast(fixed-point type=fxp<+/-,64,1> 0.0, integer=w354) -> (fixed-point=w352:fxp<+/-,64,1>)
          }
          n112 = To Double Precision Float(number=w348) -> (double precision float=w347:dbl[])
          n113 = Decimate 1D Array(w347) -> (w350:dbl[], w349:dbl[])
          n114 = Re/Im To Complex(1:w349, 2:w350) -> (0:w341:cdb[])
          n115 = Multiply(x=cdb 2.0+0.0i ("fixed-point type"), y=w341) -> (x*y=w340:cdb[])
          n116 = Array Size(array=w340) -> (size(s)=→"size(s) 1":i32)
          n117 = Enqueue Element(queue=w343, element=w340, error in (no error)=w345) -> (queue out=w342:refnum<queue>, error out=w344:errorcluster)  [unwired: 1 in, 1 out]
        }
      }
      frame True {
      }
    }
    n118 = Compound Arithmetic op=OR(w316, w323, w321) -> (w322:bool)
  }
  n119 = while {
    tunnel: w25 -> [w362]
    tunnel: w24 -> [w373]
    tunnel: w23 -> [w372]
    tunnel: w22 -> [w367]
    tunnel: w20 -> [w366]
    tunnel: [w365] -> w3
    stop <- w369 stop-if-true
    n120 = Get Queue Status(queue=w362, error in (no error)=w373) -> (queue out=w361:refnum<queue>, error out=w363:errorcluster, # elements in queue=→"# elements in queue":i32)  [unwired: 1 in, 5 out]
    n121 = Get Notifier Status(notifier=w372) -> (notifier out=w364:refnum<notifier>, current notification=w371:bool)  [unwired: 1 in, 3 out]
    n122 = case shown="False" w371 {
      tunnel: w361 -> [w392 _]
      tunnel: w363 -> [w391 w434]
      tunnel: [FALSE TRUE] -> w370
      tunnel: [w393 w434] -> w368
      tunnel: w367 -> [w382 _]
      tunnel: w366 -> [w380 _]
      tunnel: [w374 w433] -> w365
      tunnel: w364 -> [w374 w433]
      frame False {
        n123 = for {
          N: 20 -> [_]
          tunnel: w392 -> [w431]
          tunnel: [w429] -> w381 mode=concatenating
          shift-right: [w432] -> w393
          shift-left: w391 -> [w430]
          n124 = Dequeue Element(queue=w431, error in (no error)=w430) -> (element=w429:cdb[], error out=w432:errorcluster)  [unwired: 1 in, 2 out]
        }
        n125 = Array Size(array=w381) -> (size(s)=→"size(s) 2":i32)
        n126 = Reciprocal(x=w382) -> (1/x=w385:dbl)
        n127 = case shown="True" "Host decimation?" {
          tunnel: [1.0 ("total decimation") w415] -> w384
          tunnel: w381 -> [w414 w419]
          tunnel: w380 -> [_ w418]
          tunnel: [w414 w417] -> w375
          frame False {
          }
          frame True {
            n128 = call "LIA DFD Decimation.vi"("decimate by 2 times"=1, "filter in"=w418, "data in"=w419) -> ("decimated data"=w417:cdb[], "total decimation"=w415:dbl)  [unwired: 7 in]
          }
        }
        n129 = Compound Arithmetic op=MULTIPLY(w385, 256.0 ("value"), w384) -> (w378:dbl)
        n130 = Complex To Re/Im(x + iy=w375) -> (x=w389:dbl[], y=w388:dbl[])
        n131 = Array Size(array=w375) -> (size(s)=→"size(s) 3":i32)
        n132 = Bundle By Name("Y"=w375, "dt"=w378) -> (w377:waveform(cdb))  [unwired: 1 in]
        n133 = Build Array(w389, w388) -> (→"Waveform Graph 3":dbl[][])
        n134 = disable-structure shown="Disabled" {
          disable-tunnel: w377 -> [w395 _]
          frame Disabled {
            n135 = disable-structure shown="Enabled" {
              disable-tunnel: [w397 w404] -> w396
              disable-tunnel: w395 -> [w401 w412]
              frame Disabled {
                w402 = T17 1 items=["Rectangle"=0, "Hanning"=1, "Hamming"=2, "Blackman-Harris"=3, "Exact Blackman"=4, "Blackman"=5, "Flat Top"=6, "4 Term B-Harris "=7, "7 Term B-Harris"=8, "Low Sidelobe"=9, "Blackman Nuttall"=11, "Triangle"=30, "Bartlett-Hanning"=31, "Bohman"=32, "Parzen"=33, "Welch"=34, "Kaiser"=60, "Dolph-Chebyshev"=61, "Gaussian"=62] ("window")
                n136 = call "LIA Power Spectrum.vi"("window"=w402, "waveform"=w401) -> ("Waveform Graph 5"=w400:cluster{"x0":dbl, "dx":dbl, "Y":dbl[]})  [unwired: 9 in]
                n137 = call "LIA Vrms2 to dBm.vi"("Power Spectrum / PSD"=w400) -> ("output cluster"=w398:cluster{"f0":dbl, "df":dbl, "magnitude":dbl[]}, "Power Spectrum / PSD (dBm)"=w399:cluster{"f0":dbl, "df":dbl, "magnitude":dbl[]})  [unwired: 9 in]
                n138 = Build Array(w399, w398) -> (w397:cluster{"f0":dbl, "df":dbl, "magnitude":dbl[]}[])
              }
              frame Enabled {
                w405 = T16 0 items=["Power Spectrum", "Power Spectral Density"] ("export mode")
                w410 = T17 1 items=["Rectangle"=0, "Hanning"=1, "Hamming"=2, "Blackman-Harris"=3, "Exact Blackman"=4, "Blackman"=5, "Flat Top"=6, "4 Term B-Harris "=7, "7 Term B-Harris"=8, "Low Sidelobe"=9, "Blackman Nuttall"=11, "Triangle"=30, "Bartlett-Hanning"=31, "Bohman"=32, "Parzen"=33, "Welch"=34, "Kaiser"=60, "Dolph-Chebyshev"=61, "Gaussian"=62] ("window")
                n139 = call-poly <vilib>:"FFT Power Spectrum and PSD.vi"("export mode"=w405, "averaging parameters"="averaging parameters", "restart averaging (F)"="restart averaging (F)", "dB On (F)"=TRUE, "window"=w410, "time signal"=w412) -> ("Power Spectrum / PSD"=w408:cluster{"f0":dbl, "df":dbl, "magnitude":dbl[]})  [unwired: 2 in, 3 out]
                n140 = call "LIA Vrms2 to dBm.vi"("Power Spectrum / PSD"=w408) -> ("output cluster"=w403:cluster{"f0":dbl, "df":dbl, "magnitude":dbl[]}, "Power Spectrum / PSD (dBm)"=w407:cluster{"f0":dbl, "df":dbl, "magnitude":dbl[]})  [unwired: 9 in]
                n141 = Build Array(w407, w403) -> (w404:cluster{"f0":dbl, "df":dbl, "magnitude":dbl[]}[])
              }
            }
            "Power Spectrum (dBm)" <- w396
          }
          frame Enabled {
          }
        }
        n142 = disable-structure shown="Enabled" {
          disable-tunnel: w375 -> [w428 _]
          frame Enabled {
            n143 = Complex To Polar(r * e^(i*theta)=w428) -> (r=w420:dbl[])  [unwired: 1 out]
            n144 = Array Max & Min(array=w420) -> (max value=w425:dbl, min value=w424:dbl)  [unwired: 2 out]
            "lock-in.max" <- w425
            "lock-in.min" <- w424
            n145 = Build Array(w420) -> (→"Waveform Graph 4":dbl[][])
            n146 = call <vilib>:"Std Deviation and Variance.vi"("X"=w420) -> ("mean"=w421:dbl, "standard deviation"=w423:dbl)  [unwired: 1 in, 1 out]
            "lock-in.deviation" <- w423
            "lock-in.mean" <- w421
            n147 = Subtract(x=w425, y=w424) -> (x-y=→"lock-in.max-min":dbl)
            n148 = Bundle("mean"=w421, "standard deviation"=w423) -> (→"Result":cluster{"mean":dbl, "standard deviation":dbl})  [unwired: 1 in]
          }
          frame Disabled {
          }
        }
      }
      frame True {
      }
    }
    n149 = Compound Arithmetic op=OR(w370, w368) -> (w369:bool)
  }
  n150 = Send Notification(notification=TRUE, notifier=w3) -> (notifier out=w2:refnum<notifier>)  [unwired: 1 in, 1 out]
  n151 = Send Notification(notification=TRUE, notifier=w75) -> (notifier out=w73:refnum<notifier>)  [unwired: 1 in, 1 out]
  n152 = Send Notification(notification=TRUE, notifier=w78) -> (notifier out=w74:refnum<notifier>)  [unwired: 1 in, 1 out]
  n153 = flat-sequence {
    tunnel: w74 -> [w437]
    tunnel: w73 -> [_]
    tunnel: w26 -> [w436]
    tunnel: w2 -> [_]
    frame #0 {
      n154 = Release Queue(queue=w436) -> ()  [unwired: 2 in, 3 out]
      n155 = Release Notifier(notifier=w437) -> ()  [unwired: 2 in, 3 out]
    }
  }
  n156 = Merge Errors(w71, w72) -> (w70:errorcluster)
  n157 = call-dynamic "Close.vi"("error in"=w70, "host in"=w80) -> ("error out"=w64:errorcluster)  [unwired: 8 in, 1 out]
  n158 = call <vilib>:"Simple Error Handler.vi"("error in (no error)"=w64) -> ()  [unwired: 4 in, 5 out]
